vi "Heater.vi"(7 "ON":bool, 11 "Temp in":dbl) -> (3 "Temp out":dbl)   [LabVIEW 2016]
panel:
  out "Waveform Graph":dbl[](graph)
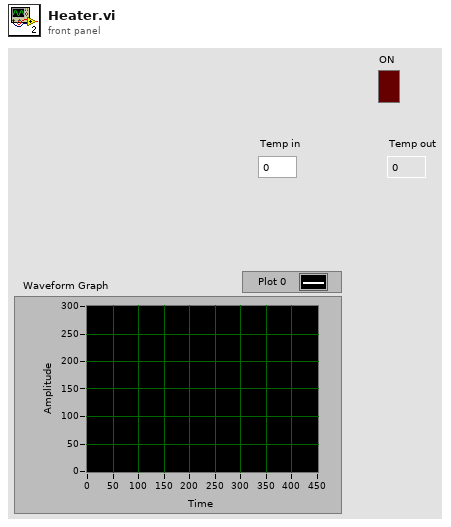
[diagram p1: front panel]
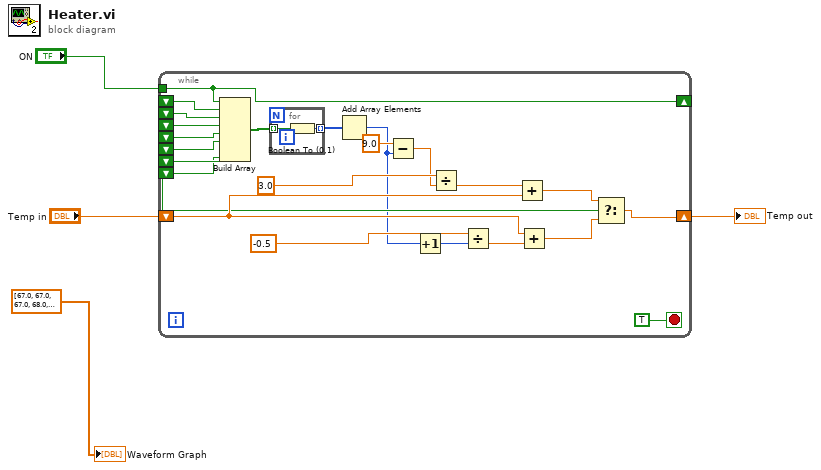
[diagram p0: block diagram]
diagram:
  n1 = while {
    shift-right: [w22] -> w2
    shift-left: "Temp in" -> [w25]
    shift-right: [w9] -> _
    shift-left: _ -> [w8]
    shift-left: _ -> [w21]
    shift-left: _ -> [w20]
    shift-left: _ -> [w19]
    shift-left: _ -> [w18]
    shift-left: _ -> [w17]
    shift-left: _ -> [w16]
    tunnel: "ON" -> [w9]
    stop <- TRUE stop-if-true
    n2 = Build Array(w9, w8, w21, w20, w19, w18, w17, w16) -> (w15:bool[])
    n3 = for {
      tunnel: w15 -> [w29] mode=indexing
      tunnel: [w28] -> w14 mode=indexing
      n4 = Boolean To (0,1)(Boolean=w29) -> (0, 1=w28:i16)
    }
    n5 = Add Array Elements(numeric array=w14) -> (sum=w6:i16)
    n6 = Subtract(x=9.0, y=w6) -> (x-y=w11:dbl)
    n7 = Increment(x=w6) -> (x+1=w5:i16)
    n8 = Divide(x=3.0, y=w11) -> (x/y=w13:dbl)
    n9 = Divide(x=-0.5 ("y"), y=w5) -> (x/y=w12:dbl)
    n10 = Add(x=w13, y=w25) -> (x+y=w26:dbl)
    n11 = Add(x=w25, y=w12) -> (x+y=w23:dbl)
    n12 = Select(t=w26, s=w8, f=w23) -> (s? t:f=w22:dbl)
  }
  "Temp out" <- w2
  "Waveform Graph" <- dbl[] [67.0, 67.0, 67.0, 68.0, 68.0, 68.0, 68.0, 68.0, 68.0, 69.0, 69.0, 70.0, 70.0, 72.0, 73.0, 74.0, 76.0, 78.0, 80.0, 82.0, 84.0, 87.0, 89.0, 92.0, 95.0, 98.0, 101.0, 105.0, 108.0, 113.0, 117.0, 121.0, 125.0, 129.0, 134.0, 138.0, 143.0, 148.0, 152.0, 156.0, 159.0, 162.0, 165.0, 167.0, 169.0, 171.0, 172.0, 173.0, 174.0, 175.0, 176.0, 177.0, 177.0, 177.0, 178.0, 179.0, 179.0, 179.0, 179.0, 179.0, 179.0, 180.0, 179.0, 179.0, 179.0, 179.0, 179.0, 179.0, 178.0, 178.0, 178.0, 177.0, 177.0, 176.0, 176.0, 175.0, 175.0, 174.0, 174.0, 173.0, 173.0, 172.0, 172.0, 171.0, 171.0, 170.0, 169.0, 169.0, 168.0, 167.0, 167.0, 166.0, 166.0, 165.0, 165.0, 164.0, 164.0, 163.0, 162.0, 162.0, 161.0, 160.0, 160.0, 159.0, 159.0, 158.0, 157.0, 157.0, 156.0, 156.0, 155.0, 155.0, 154.0, 154.0, 153.0, 153.0, 152.0, 151.0, 151.0, 150.0, 150.0, 149.0, 149.0, 148.0, 148.0, 147.0, 146.0, 146.0, 145.0, 145.0, 144.0, 144.0, 143.0, 143.0, 142.0, 142.0, 141.0, 140.0, 140.0, 140.0, 139.0, 139.0, 138.0, 138.0, 137.0, 137.0, 137.0, 138.0, 138.0, 139.0, 140.0, 141.0, 143.0, 144.0, 145.0, 146.0, 147.0, 148.0, 149.0, 150.0, 151.0, 151.0, 152.0, 152.0, 152.0, 153.0, 153.0, 153.0, 153.0, 153.0, 153.0, 153.0, 153.0, 153.0, 153.0, 153.0, 153.0, 153.0, 153.0, 153.0, 153.0, 153.0, 154.0, 155.0, 157.0, 158.0, 161.0, 162.0, 165.0, 167.0, 170.0, 173.0, 176.0, 179.0, 183.0, 186.0, 189.0, 193.0, 197.0, 201.0, 205.0, 208.0, 212.0, 216.0, 220.0, 224.0, 228.0, 232.0, 236.0, 239.0, 242.0, 244.0, 246.0, 248.0, 250.0, 251.0, 252.0, 252.0, 253.0, 253.0, 253.0, 253.0, 252.0, 252.0, 252.0, 251.0, 251.0, 250.0, 249.0, 248.0, 247.0, 247.0, 246.0, 245.0, 244.0, 243.0, 242.0, 241.0, 240.0, 238.0, 237.0, 236.0, 235.0, 234.0, 233.0, 232.0, 230.0, 230.0, 229.0, 227.0, 226.0, 225.0, 224.0, 224.0, 224.0, 224.0, 224.0, 225.0, 226.0, 227.0, 228.0, 231.0, 233.0, 235.0, 236.0, 238.0, 239.0, 240.0, 241.0, 241.0, 242.0, 242.0, 242.0, 242.0, 241.0, 241.0, 241.0, 241.0, 240.0, 239.0, 239.0, 238.0, 238.0, 237.0, 236.0, 235.0, 234.0, 233.0, 232.0, 231.0, 230.0, 229.0, 228.0, 228.0, 227.0, 226.0, 225.0, 226.0, 226.0, 226.0, 227.0, 227.0, 227.0, 226.0, 226.0, 226.0, 225.0, 225.0, 225.0, 224.0, 224.0, 223.0, 223.0, 222.0, 222.0, 221.0, 220.0, 219.0, 219.0, 218.0, 217.0, 217.0, 216.0, 211.0, 199.0, 187.0, 176.0, 167.0, 161.0, 153.0, 138.0, 126.0, 117.0, 108.0, 99.0, 94.0, 90.0, 86.0, 83.0, 81.0, 79.0, 77.0, 75.0, 74.0, 73.0, 72.0, 71.0, 70.0, 69.0, 69.0, 68.0, 67.0, 67.0, 66.0, 66.0, 65.0, 64.0, 64.0, 63.0, 62.0, 62.0, 61.0, 61.0, 61.0, 37.0, 28.0, 60.0, 60.0, 60.0, 60.0, 59.0, 59.0, 59.0, 58.0, 58.0, 57.0, 57.0, 57.0, 56.0, 56.0, 55.0, 55.0, 55.0, 54.0, 54.0, 54.0, 53.0, 53.0, 53.0, 53.0, 52.0, 52.0, 52.0, 51.0, 51.0, 51.0, 51.0, 51.0, 50.0, 50.0, 50.0, 50.0, 49.0, 49.0, 49.0, 49.0, 49.0, 49.0, 49.0, 48.0, 48.0, 48.0, 48.0, 48.0, 48.0] ("History Data")
